vi "read_data.vi"() -> ()   [LabVIEW 2020]
panel:
  out "数据":dbl[](array[numeric])
  in  "文件路径（使用对话框）":path
  out "从文件中读取的数据":dbl[](graph)
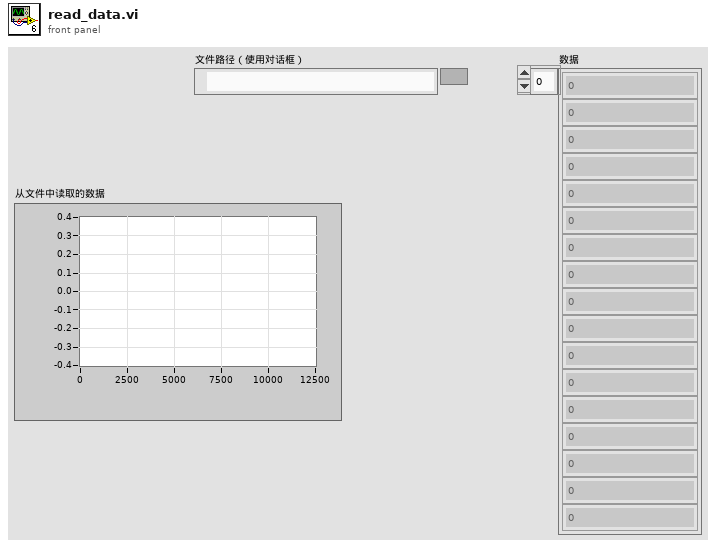
[diagram p1: front panel]
types:
  T1 = enum16{"open", "replace", "create", "open or create", "replace or create", "replace or create with confirmation"}
  T2 = enum16{"big-endian, network order", "native, host order", "little-endian"}
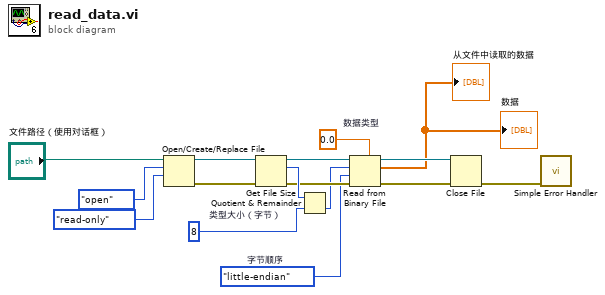
[diagram p0: block diagram]
diagram:
  w6 = T2."little-endian"  # 字节顺序
  w8 = i64 8  # 类型大小（字节）
  w9 = 0.0  # 数据类型
  n1 = Open/Create/Replace File(file path (use dialog)="文件路径（使用对话框）", operation (0:open)=T1."open", access (0:read/write)=enum16{"read/write", "read-only", "write-only"}."read-only") -> (refnum out=w3:refnum<file>, error out=w4:errorcluster)  [unwired: 3 in, 1 out]
  n2 = Get File Size(file=w3, error in=w4) -> (refnum out=w16:refnum<file>, size (in bytes)=w13:i64, 0:w12:errorcluster)
  n3 = Quotient & Remainder(x=w13, y=w8) -> (floor(x/y)=w7:i64)  [unwired: 1 out]
  n4 = Read from Binary File(5:w9, 8:w12, 9:w6, 10:w7, 11:w16) -> (0:w14:errorcluster, 2:→"从文件中读取的数据" →"数据":dbl[], 3:w15:refnum<file>)  [unwired: 1 in, 1 out]
  n5 = Close File(refnum=w15, error in=w14) -> (error out=w2:errorcluster)  [unwired: 1 out]
  n6 = call <vilib>:"Simple Error Handler.vi"("error in (no error)"=w2) -> ()  [unwired: 4 in, 5 out]
